vi "Open SystemLink Connection.vi"   [LabVIEW 2025, in "SystemLink_Repo_API.lvlib"]
uses:
  SystemLink_Repo_API.lvlib
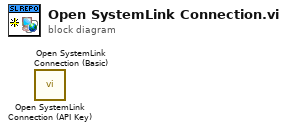
[diagram p0: block diagram]
diagram:
  n1 = call "Open SystemLink Connection (API Key).vi"() -> ()  [unwired: 14 in, 2 out]
  n2 = call "Open SystemLink Connection (Basic).vi"() -> ()  [unwired: 14 in, 2 out]
